vi "Digital Tach.vi"(1 "Input Pin":refnum<k21>) -> (0 "Tach Ticks":u32)   [LabVIEW 2019]
uses:
  <vilib>/rvi/eio/common/nirviEmuTemplateMethod_errors.vi
  <vilib>/eio/EIONode/EIONode.xnode
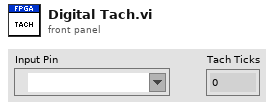
[diagram p1: front panel]
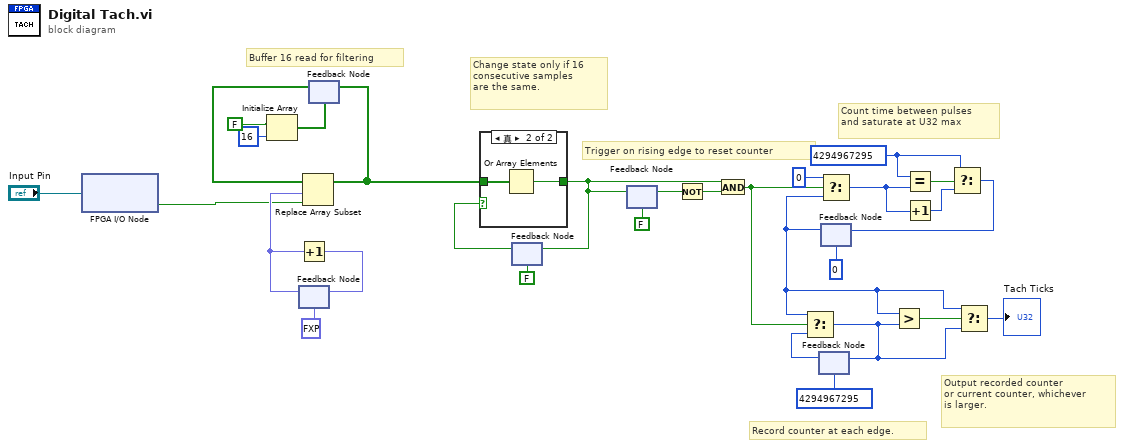
[diagram p0: block diagram]
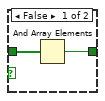
[diagram p2: hidden frame]
diagram:
  w7 = u32 4294967295
  # "Output recorded counter\nor current counter, whichever\nis larger."
  # "Record counter at each edge."
  # "Count time between pulses\nand saturate at U32 max"
  # "Change state only if 16\nconsecutive samples\nare the same."
  # "Trigger on rising edge to reset counter"
  # "Buffer 16 read for filtering"
  n1 = xnode "FPGA I/O Node"("FPGA I/O输入"="Input Pin") -> ("I/O项"=w22:bool)  [unwired: 1 out]
  n2 = Initialize Array(FALSE, 16 ("dimension size")) -> (w25:bool[])
  n3 = feedback #1(fxp<+,4,4> 0.0) -> (w23:fxp<+,4,4>)
  n4 = Increment(x=w23) -> (x+1=w28:fxp<+,4,4>)
  n5 = feedback-in #1(w28) -> ()
  n6 = feedback #2(w25) -> (w24:bool[])
  n7 = Replace Array Subset(array=w24, new element=w22, index=w23) -> (w19:bool[])
  n8 = feedback-in #2(w19) -> ()
  n9 = feedback #3(FALSE) -> (w20:bool)
  n10 = case shown="真" w20 {
    tunnel: w19 -> [w32 w34]
    tunnel: [w31 w33] -> w15
    frame False {
      n11 = And Array Elements(Boolean array=w32) -> (logical AND=w31:bool)
    }
    frame True {
      n12 = Or Array Elements(Boolean array=w34) -> (logical OR=w33:bool)
    }
  }
  n13 = feedback-in #3(w15) -> ()
  n14 = feedback-in #4(w15) -> ()
  n15 = feedback #4(FALSE) -> (w17:bool)
  n16 = Not(x=w17) -> (.not. x?=w16:bool)
  n17 = And(x=w15, y=w16) -> (x .and. y?=w11:bool)
  n18 = feedback #5(u32 4294967295) -> (w10:u32)
  n19 = feedback #6(u32 0) -> (w3:u32)
  n20 = Select(t=w3, s=w11, f=w10) -> (s? t:f=w2:u32)
  n21 = feedback-in #5(w2) -> ()
  n22 = Select(t=u32 0, s=w11, f=w3) -> (s? t:f=w9:u32)
  n23 = Greater?(x=w3, y=w2) -> (0:w4:bool)
  n24 = Equal?(x=w7, y=w9) -> (x = y?=w8:bool)
  n25 = Increment(x=w9) -> (x+1=w6:u32)
  n26 = Select(t=w7, s=w8, f=w6) -> (s? t:f=w5:u32)
  n27 = feedback-in #6(w5) -> ()
  n28 = Select(t=w3, s=w4, f=w2) -> (s? t:f=→"Tach Ticks":u32)
